vi "保存数据格式.vi"(4 "Name":string, 5 "Path":path, 8 "数据":dynamicdata(waveform), 10 "ID":u8 format="%x", 11 "是否保存":bool) -> ()   [LabVIEW 2016]
uses:
  <vilib>/Utility/file.llb/Write Delimited Spreadsheet (DBL).vi
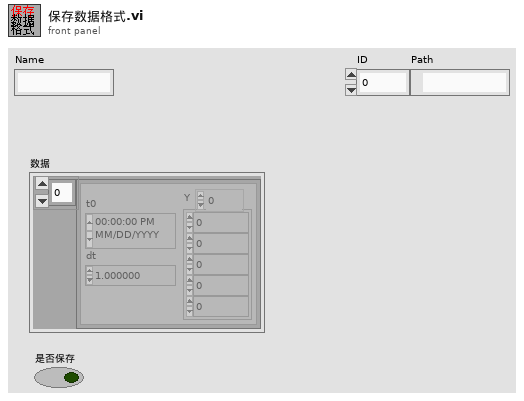
[diagram p1: front panel]
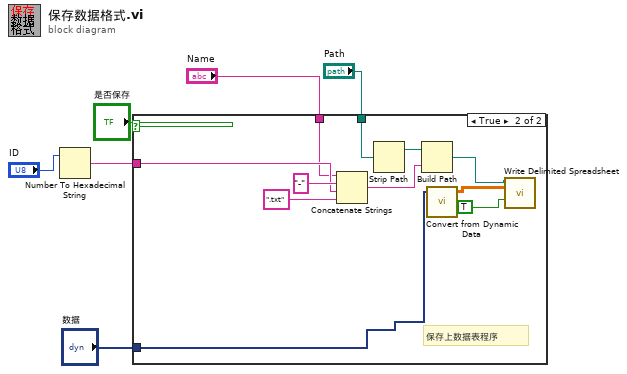
[diagram p0: block diagram]
diagram:
  n1 = Number To Hexadecimal String(2:"ID") -> (0:w3:string)  [unwired: 1 in]
  n2 = case shown="True" "是否保存" {
    tunnel: "数据" -> [_ w7]
    tunnel: w3 -> [_ w11]
    tunnel: "Path" -> [_ w10]
    tunnel: "Name" -> [_ w8]
    frame False {
    }
    frame True {
      # "保存上数据表程序"
      n3 = Concatenate Strings(w8, "-" ("字符串"), w11, ".txt" ("字符串")) -> (w15:string)
      n4 = Strip Path(path=w10) -> (stripped path=w17:path)  [unwired: 1 out]
      n5 = Build Path(base path=w17, name or relative path=w15) -> (appended path=w14:path)
      n6 = call "Convert from Dynamic Data"("Dynamic Data Type"=w7) -> ("Array"=w12:dbl[][])  [unwired: 3 in]
      n7 = call-poly <vilib>:"Write Delimited Spreadsheet.vi"("file path (dialog if empty)"=w14, "2D data"=w12, "append to file? (new file:F)"=TRUE) -> ()  [unwired: 11 in, 2 out]
    }
  }
